vi "tm481_wview.vi"() -> ()   [LabVIEW 2011]
panel:
  in  "Exposure B":dbl=0.01
  in  "Exposure A":dbl=0.04 format="%#_6f"
  out "Current Timestamp":dbl
  out "Image B":u16[][](graph) caption="Image"
  out "Image A":u16[][](graph) caption="Image"
  in  "Vertical Width":i32=512
  in  "Horizontal Width":i32=1024
  in  "Vertical Offset B":i32=64
  in  "Horizontal Offset B":i32=256
  in  "Vertical Offset A":i32=128
  in  "Horizontal Offset A":i32=512
  out "Frames Per Second":dbl
  in  "Quit":bool
  out "Error Out":errorcluster {"code" format="%.0x"}
  # "This is just a simple example\nof how to setup a camera for\na W-View application with\na Flash4.0 LT"
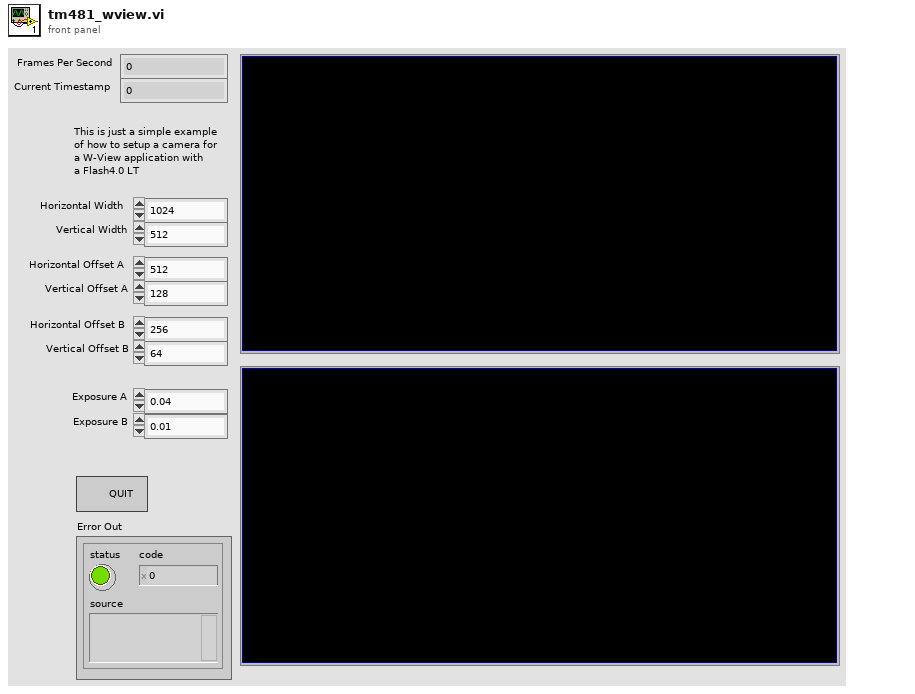
[diagram p1: front panel]
types:
  T1 = cluster{"Horizontal Offset A":i32, "Vertical Offset A":i32, "Horizontal Offset B":i32, "Vertical Offset B":i32, "Horizontal Width":i32, "Vertical Width":i32}
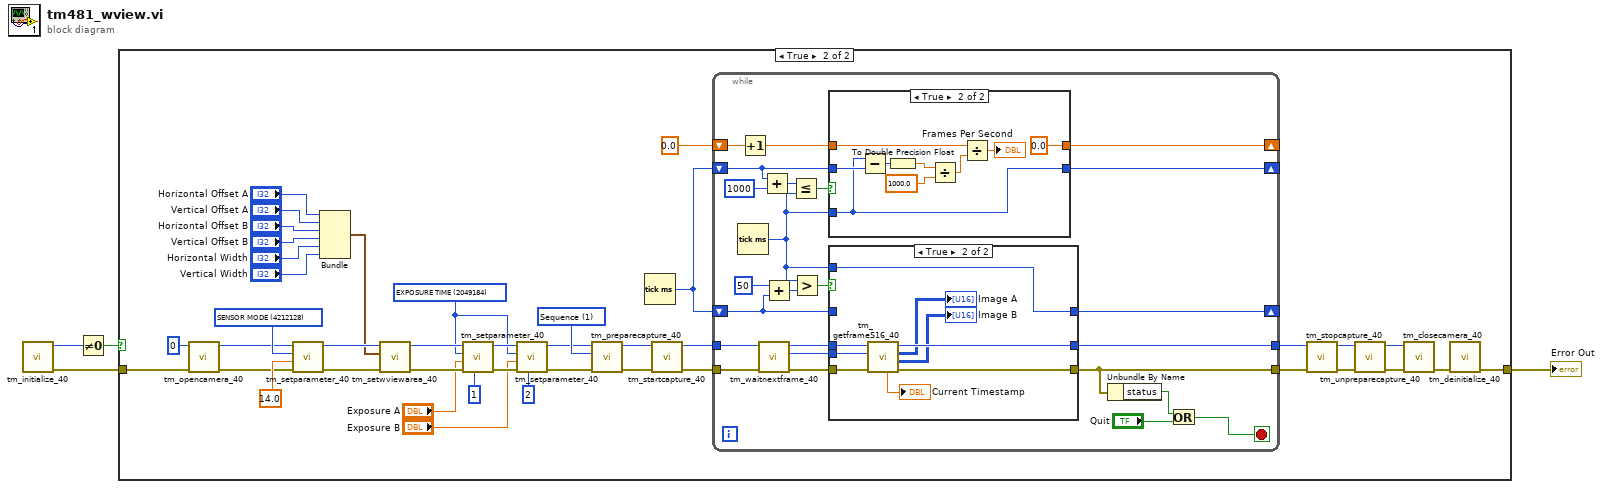
[diagram p0: block diagram]
diagram:
  n1 = call <userlib>:"tm_initialize_40.vi"() -> ("error out"=w1:errorcluster, "Number Of Cameras"=w2:u32)  [unwired: 8 in, 2 out]
  n2 = Not Equal To 0?(x=w2) -> (x != 0?=w4:bool)
  n3 = case shown="True" w4 {
    tunnel: w1 -> [w5 w46]
    tunnel: [w5 w43] -> w3
    frame False {
    }
    frame True {
      w6 = u32 2049184 items=["SENSOR MODE"=4212128, "READOUT SPEED"=4211872, "READOUT DIRECTION"=4211904, "TRIGGER GLOBAL EXPOSURE"=2049680, "TRIGGER DELAY"=1066480, "INTERNAL TRIGGER HANDLING"=1066496, "SYNC READOUT SYSTEM BLANK"=1066528, "SENSOR TEMPERATURE"=2115232, "SENSOR COOLER STATUS"=2115280, "EXPOSURE TIME"=2049184, "DEFECT CORRECT MODE"=4670368, "BINNING"=4215968, "INTERNAL LINE SPEED"=4226000, "INTERNAL LINE INTERVAL"=4226016, "NUMBER OF OUTPUT TRIGGER CONNECTOR"=1852320, "OUTPUT TRIGGER SOURCE[0]"=1852576, "OUTPUT TRIGGER SOURCE[1]"=1852832, "OUTPUT TRIGGER SOURCE[2]"=1853088, "OUTPUT TRIGGER POLARITY[0]"=1852592, "OUTPUT TRIGGER POLARITY[1]"=1852848, "OUTPUT TRIGGER POLARITY[2]"=1853104, "OUTPUT TRIGGER ACTIVE[0]"=1852608, "OUTPUT TRIGGER ACTIVE[1]"=1852864, "OUTPUT TRIGGER ACTIVE[2]"=1853120, "OUTPUT TRIGGER DELAY[0]"=1852624, "OUTPUT TRIGGER DELAY[1]"=1852880, "OUTPUT TRIGGER DELAY[2]"=1853136, "OUTPUT TRIGGER PERIOD[0]"=1852640, "OUTPUT TRIGGER PERIOD[1]"=1852896, "OUTPUT TRIGGER PERIOD[2]"=1853152, "OUTPUT TRIGGER KIND[0]"=1852656, "OUTPUT TRIGGER KIND[1]"=1852912, "OUTPUT TRIGGER KIND[2]"=1853168, "OUTPUT TRIGGER BASE SENSOR[0]"=1852672, "OUTPUT TRIGGER BASE SENSOR[1]"=1852928, "OUTPUT TRIGGER BASE SENSOR[2]"=1853184, "OUTPUT TRIGGER PRE HSYNC COUNT"=1852704] ("Parameter")
      w28 = u32 4212128 items=["SENSOR MODE"=4212128, "CCD MODE"=4212384, "READOUT MODE"=4211872, "ACTIVE VIEW INDEX"=4343136, "BITS PER CHANNEL"=4342976, "IMAGE PIXEL TYPE"=4343296, "BINNING"=4215968, "EXPOSURE TIME"=2049184, "CONTRAST GAIN"=3163312, "CONTRAST OFFSET"=3163328, "LIGHT MODE"=2114720, "SENSITIVITY"=2114992, "PHOTON IMAGING MODE"=2115200, "HIGH DYNAMIC RANGE MODE"=3163360, "WHITE BALANCE"=3163568, "TEMPERATURE"=2115232, "TEMPERATURE TARGET"=2115264, "SENSOR COOLER FAN"=2115296, "LINEBUNDLE HEIGHT"=4212192, "MECHANICAL SHUTTER"=2115488, "BACK FOCUS POSITION"=8422304, "TRIGGER CONNECTOR"=1066432, "TRIGGER SOURCE"=1066144, "OUTPUT TRIGGER SOURCE"=1852576, "TRIGGER GLOBAL EXPOSURE"=2049680, "FIRST TRIGGER BEHAVIOR"=2049696, "CHANNEL SYNC"=1852352, "READOUT DIRECTION"=4211904, "PRE HSYNC COUNT"=1852704, "INTERNAL LINE SPEED"=4191408, "INTERNAL LINE INTERVAL"=4191424] ("Parameter")
      w34 = 1 items=["Snap", "Sequence"] ("Capture mode")
      n4 = call <userlib>:"tm_opencamera_40.vi"("error in (no error)"=w46, "Camera Index"=u32 0) -> ("error out"=w26:errorcluster, "Handle out"=w27:u32)  [unwired: 7 in, 1 out]
      n5 = call <userlib>:"tm_setparameter_40.vi"("error in (no error)"=w26, "Value in"=14.0, "Parameter"=w28, "Handle in"=w27) -> ("error out"=w24:errorcluster, "Handle out"=w25:u32)  [unwired: 6 in]
      n6 = Bundle("Horizontal Offset A"="Horizontal Offset A", "Vertical Offset A"="Vertical Offset A", "Horizontal Offset B"="Horizontal Offset B", "Vertical Offset B"="Vertical Offset B", "Horizontal Width"="Horizontal Width", "Vertical Width"="Vertical Width") -> (w23:T1)  [unwired: 1 in]
      n7 = call <userlib>:"tm_setwviewarea_40.vi"("error in (no error)"=w24, "Sub Region"=w23, "Handle in"=w25) -> ("error out"=w15:errorcluster, "Handle out"=w16:u32)  [unwired: 7 in]
      n8 = call <userlib>:"tm_setparameter_40.vi"("Index"=1, "error in (no error)"=w15, "Value in"="Exposure A", "Parameter"=w6, "Handle in"=w16) -> ("error out"=w13:errorcluster, "Handle out"=w14:u32)  [unwired: 5 in]
      n9 = call <userlib>:"tm_setparameter_40.vi"("Index"=2, "error in (no error)"=w13, "Value in"="Exposure B", "Parameter"=w6, "Handle in"=w14) -> ("error out"=w12:errorcluster, "Handle out"=w11:u32)  [unwired: 5 in]
      n10 = call <userlib>:"tm_preparecapture_40.vi"("error in (no error)"=w12, "Capture mode"=w34, "Handle in"=w11) -> ("error out"=w32:errorcluster, "Handle out"=w33:u32)  [unwired: 5 in, 2 out]
      n11 = Tick Count (ms)() -> (millisecond timer value=w30:u32)
      n12 = call <userlib>:"tm_startcapture_40.vi"("error in (no error)"=w32, "Handle in"=w33) -> ("error out"=w35:errorcluster, "Handle out"=w36:u32)  [unwired: 8 in]
      n13 = while {
        tunnel: [w49] -> w39
        tunnel: [w50] -> w40
        tunnel: w36 -> [w67]
        tunnel: w35 -> [w68]
        shift-right: [w65] -> _
        shift-left: w30 -> [w62]
        shift-right: [w66] -> _
        shift-left: 0.0 -> [w59]
        shift-right: [w48] -> _
        shift-left: w30 -> [w51]
        stop <- w47 stop-if-true
        n14 = Tick Count (ms)() -> (millisecond timer value=w52:u32)
        n15 = Increment(x=w59) -> (x+1=w60:dbl)
        n16 = call <userlib>:"tm_waitnextframe_40.vi"("error in (no error)"=w68, "Handle in"=w67) -> ("error out"=w57:errorcluster, "Frame Index"=w56:i32, "Handle out"=w58:u32)  [unwired: 6 in, 1 out]
        n17 = Add(x=w62, y=u32 1000) -> (x+y=w64:u32)
        n18 = Add(x=u32 50, y=w51) -> (x+y=w54:u32)
        n19 = Less Or Equal?(x=w64, y=w52) -> (x <= y?=w61:bool)
        n20 = Greater?(x=w52, y=w54) -> (0:w53:bool)
        n21 = case shown="True" w61 {
          tunnel: w62 -> [w84 w87]
          tunnel: [w84 w85] -> w65
          tunnel: w60 -> [w83 w91]
          tunnel: w52 -> [_ w85]
          tunnel: [w83 0.0] -> w66
          frame False {
          }
          frame True {
            n22 = Subtract(x=w85, y=w87) -> (x-y=w86:u32)
            n23 = To Double Precision Float(number=w86) -> (double precision float=w93:dbl)
            n24 = Divide(x=w93, y=1000.0) -> (x/y=w90:dbl)
            n25 = Divide(x=w91, y=w90) -> (x/y=→"Frames Per Second":dbl)
          }
        }
        n26 = case shown="True" w53 {
          tunnel: w58 -> [w73 w79]
          tunnel: w57 -> [w72 w81]
          tunnel: w56 -> [_ w80]
          tunnel: w51 -> [w71 _]
          tunnel: w52 -> [_ w82]
          tunnel: [w73 w78] -> w49
          tunnel: [w72 w75] -> w50
          tunnel: [w71 w82] -> w48
          frame False {
          }
          frame True {
            n27 = call <userlib>:"tm_getframeS16_40.vi"("error in (no error)"=w81, "Frame Index"=w80, "Handle in"=w79) -> ("error out"=w75:errorcluster, "Data B"=→"Image B":u16[][], "Data A"=→"Image A":u16[][], "Handle out"=w78:u32, "Timestamp"=→"Current Timestamp":dbl)  [unwired: 4 in]
          }
        }
        n28 = Unbundle By Name(w50) -> ("status"=w70:bool)
        n29 = Or(x=w70, y="Quit") -> (x .or. y?=w47:bool)
      }
      n30 = call <userlib>:"tm_stopcapture_40.vi"("error in (no error)"=w40, "Handle in"=w39) -> ("error out"=w37:errorcluster, "Handle out"=w38:u32)  [unwired: 8 in]
      n31 = call <userlib>:"tm_unpreparecapture_40.vi"("error in (no error)"=w37, "Handle in"=w38) -> ("error out"=w42:errorcluster, "Handle out"=w41:u32)  [unwired: 8 in]
      n32 = call <userlib>:"tm_closecamera_40.vi"("error in (no error)"=w42, "Handle in"=w41) -> ("error out"=w44:errorcluster)  [unwired: 9 in]
      n33 = call <userlib>:"tm_deinitialize_40.vi"("error in (no error)"=w44) -> ("error out"=w43:errorcluster)  [unwired: 10 in]
    }
  }
  "Error Out" <- w3
